vi "Tektronix 7000 Series Acquire Continuous Waveform.vi"() -> ()   [LabVIEW 2015]
doc: "Demonstrates how to set up an oscilloscope automatically. You can configure this VI to acquire waveforms continuously from a single channel by following the following steps:\n\n1. Specify a valid VISA resource to use. \n2. Specify a channel. \n3. Specify a time-out value for reading a waveform.\n4. Run this VI. The <B>Waveform Graph</B> displays the waveform you acquire."
uses:
  Public/Data/Read (Single Waveform).vi
  Tektronix 7000 Series.lvlib
panel:
  out "Waveform Graph":waveform(dbl)(graph)
  in  "Maximum Time (10000 ms)":u32=10000
  in  "Channel (0: Channel 1)":u16(ring) format="%#_5f" items=["Channel 1", "Channel 2", "Channel 3", "Channel 4"]
  in  "Probe Attenuation (10.0)":dbl=10.0
  in  "stop":bool
  in  "VISA Resource Name":refnum<visa-resource-name>
  # "(c) 2006 - 2016 National Instruments Corporation.  ALL RIGHTS RESERVED."
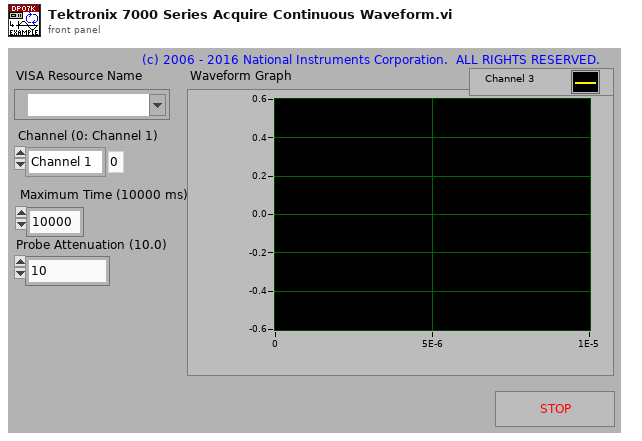
[diagram p1: front panel]
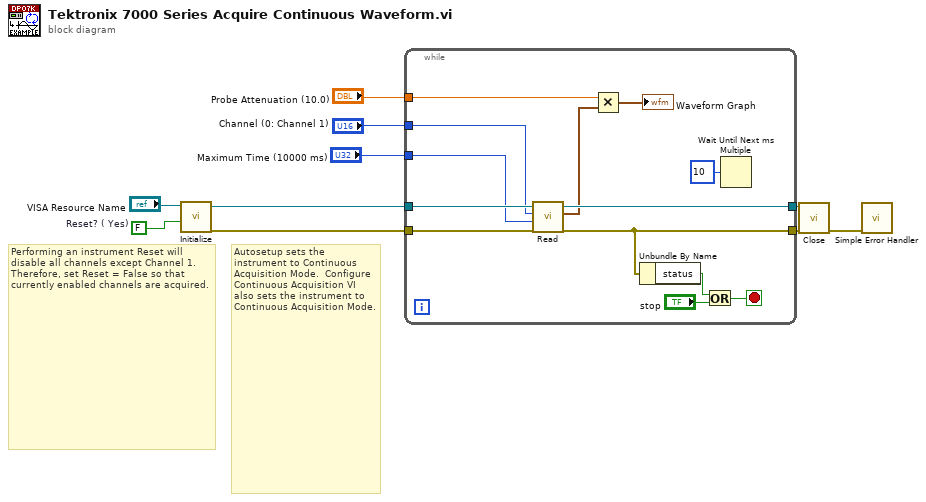
[diagram p0: block diagram]
diagram:
  w3 = FALSE  # Reset? ( Yes)
  # "Performing an instrument Reset will disable all channels except Channel 1. Therefore, set Reset = False so that currently enabled channels are acquired."
  # "Autosetup sets the instrument to Continuous Acquisition Mode.  Configure Continuous Acquisition VI also sets the instrument to Continuous Acquisition Mode."
  n1 = call "Initialize.vi"("Reset? ( Yes)"=w3, "VISA resource name"="VISA Resource Name") -> ("error out"=w1:errorcluster, "VISA resource name out"=w2:refnum<visa-resource-name>)  [unwired: 8 in]
  n2 = while {
    tunnel: w2 -> [w17]
    tunnel: w1 -> [w16]
    tunnel: "Channel (0: Channel 1)" -> [w15]
    tunnel: [w18] -> w10
    tunnel: [w19] -> w9
    tunnel: "Probe Attenuation (10.0)" -> [w12]
    tunnel: "Maximum Time (10000 ms)" -> [w11]
    stop <- w20 stop-if-true
    n3 = call-poly "Read.vi"("error in (no error)"=w16, "Maximum Time (10000 ms)"=w11, "Channel (0: Channel 1)"=w15, "VISA resource name"=w17) -> ("error out"=w19:errorcluster, "Waveform Data"=w14:waveform(dbl), "VISA resource name out"=w18:refnum<visa-resource-name>)  [unwired: 5 in]
    n4 = Multiply(x=w12, y=w14) -> (x*y=→"Waveform Graph":waveform(dbl))
    n5 = Unbundle By Name(w19) -> ("status"=w22:bool)
    n6 = Or(x=w22, y="stop") -> (x .or. y?=w20:bool)
    n7 = Wait Until Next ms Multiple(millisecond multiple=u32 10) -> ()  [unwired: 1 out]
  }
  n8 = call "Close.vi"("error in (no error)"=w9, "VISA resource name"=w10) -> ("error out"=w8:errorcluster)  [unwired: 9 in]
  n9 = call <vilib>:"Simple Error Handler.vi"("error in (no error)"=w8) -> ()  [unwired: 4 in, 5 out]
